vi "Edge Detection.vi"(8 "error in (no error)":errorcluster, 9 "File Path of Calibrated Image":path=path "C:/Users/user/Desktop/Studienarbeit Image Processing/Images Captured/Calibration/Calibration_Target  Grid Distortion_Dot Dia_1mm/Template_Calibrated Image_Exposure_950.png", 10 "Image From Camera":T1, 11 "Select the Pin to be measured":enum16{"1", "2", "3", "4", "5"}(ring)) -> (0 "error out":errorcluster, 2 "Pixel Column of the edge":sgl, 3 "Image":T1(plugin-control))   [LabVIEW 2016]
uses:
  <vilib>/vision/Measure.llb/Edge New.ctl
  <vilib>/vision/Image Controls.llb/IMAQ Image.ctl
  <vilib>/vision/NI_Vision_Development_Module.lvlib
panel:
  out "Edge Information":T2[](array[typedef]) {"Distance (Real-World)" format="%.2f"; "Location (Real-World)"."Y" format="%.2g"; "Location (Real-World)"."X" format="%.2f"; "Noise" format="%.2f"; "Location (Pixel)"."Y" format="%.2g"; "Location (Pixel)"."X" format="%.2f"; "Strength" format="%.2f"; "Distance (Pixel)" format="%.2f"}
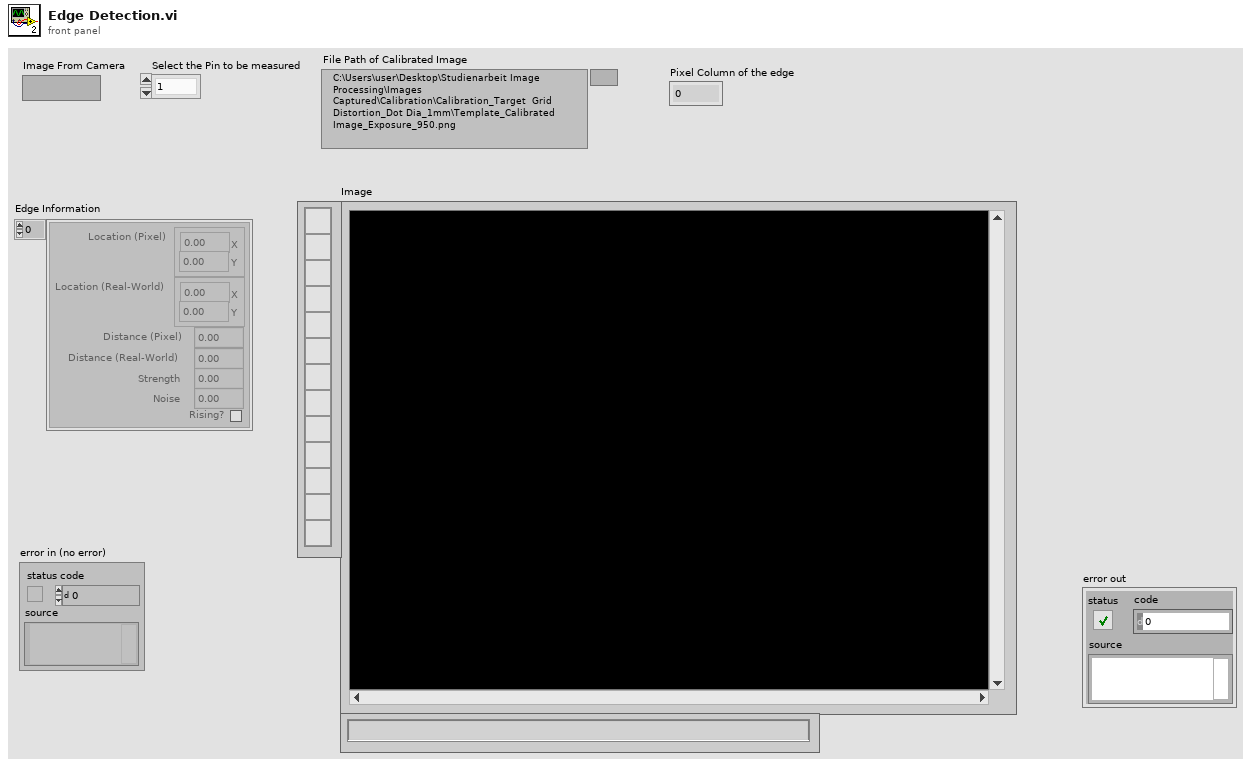
[diagram p1: front panel]
types:
  T1 = typedef "IMAQ Image.ctl" = refnum<image>
  T2 = typedef "Edge New.ctl" = cluster{"Location (Pixel)":cluster{"X":sgl, "Y":sgl}, "Location (Real-World)":cluster{"X":sgl, "Y":sgl}, "Distance (Pixel)":dbl, "Distance (Real-World)":dbl, "Strength":dbl, "Noise":dbl, "Rising?":bool}
  T3 = typedef "ROI Descriptor" = cluster{"Global Rectangle":i32[], "Contours":cluster{"ID":enum32{"External", "Internal"}, "Type":u32, "Coordinates":i32[]}[]}
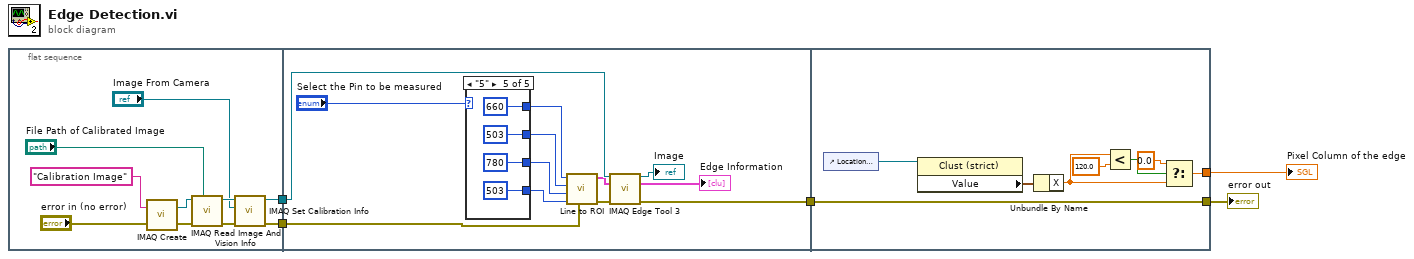
[diagram p0: block diagram]
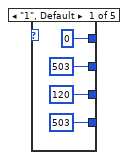
[diagram p2: hidden frame]
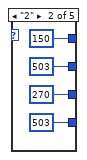
[diagram p3: hidden frame]
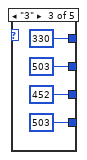
[diagram p4: hidden frame]
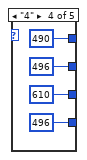
[diagram p5: hidden frame]
diagram:
  n1 = flat-sequence {
    tunnel: [w11] -> w5
    tunnel: [w10] -> w4
    tunnel: w5 -> [w20]
    tunnel: w4 -> [w26]
    tunnel: [w25] -> w3
    tunnel: [w55] -> w2
    tunnel: w3 -> [w55]
    tunnel: [w48] -> w1
    frame #0 {
      n2 = call "IMAQ Create"("Image Name"="Calibration Image", "error in (no error)"="error in (no error)") -> ("New Image"=w14:T1, "error out"=w6:errorcluster)  [unwired: 3 in]
      n3 = call "IMAQ Read Image And Vision Info"("File Path"="File Path of Calibrated Image", "error in (no error)"=w6, "Image"=w14) -> ("error out"=w8:errorcluster, "Image Out"=w12:T1)  [unwired: 6 in, 1 out]
      n4 = call "IMAQ Set Calibration Info"("error in (no error)"=w8, "Image Dst"="Image From Camera", "Image Src"=w12) -> ("error out"=w11:errorcluster, "Calibrated Image"=w10:T1)  [unwired: 7 in]
    }
    frame #1 {
      n5 = case shown="\"5\"" "Select the Pin to be measured" {
        tunnel: [0 150 ("Start X") 330 ("Start X") 490 ("Start X") 660 ("Start X")] -> w19
        tunnel: [503 503 ("Start X") 503 ("Start X") 496 ("Start X") 503 ("Start X")] -> w18
        tunnel: [120 270 ("Start X") 452 ("Start X") 610 ("Start X") 780 ("Start X")] -> w17
        tunnel: [503 503 ("Start X") 503 ("Start X") 496 ("Start X") 503 ("Start X")] -> w16
        frame "1", Default {
        }
        frame "2" {
        }
        frame "3" {
        }
        frame "4" {
        }
        frame "5" {
        }
      }
      n6 = call "Line to ROI.vi"("error in (no error)"=w20, "End Y"=w16, "End X"=w17, "Start Y"=w18, "Start X"=w19) -> ("error out"=w22:errorcluster, "ROI Descriptor"=w21:T3)  [unwired: 5 in]
      n7 = call "IMAQ Edge Tool 3"("Image"=w26, "ROI Descriptor"=w21, "error in (no error)"=w22) -> ("Image (duplicate)"=→"Image":T1, "Edge Information"=→"Edge Information":T2[], "error out"=w25:errorcluster)  [unwired: 8 in, 2 out]
    }
    frame #2 {
      n8 = control-ref of="Location (Pixel)"() -> (w49:refnum<vi>)
      n9 = property class="Clust (strict)"(reference=w49) -> ("Value"=w50:cluster{"X":sgl, "Y":sgl})  [unwired: 1 in, 2 out]
      n10 = Unbundle By Name(w50) -> ("X"=w53:sgl)
      n11 = Less?(x=w53, y=sgl 120.0) -> (x < y?=w52:bool)
      n12 = Select(t=sgl 0.0, s=w52, f=w53) -> (s? t:f=w48:sgl)
    }
  }
  "error out" <- w2
  "Pixel Column of the edge" <- w1
